vi "Write Retry on Timeout.vi"(8 "error in (no error)":errorcluster, 10 "Retry on Timeout":bool, 11 "CIFFIFO in":refnum<class "CIFfifo.lvclass">) -> (0 "error out":errorcluster, 3 "CIFFIFO out":refnum<class "CIFfifo.lvclass">)   [LabVIEW 2021, in "CIFfifo.lvclass"]
uses:
  CIFfifo.lvclass
  CIFfifo.lvclass/CIFfifo.ctl
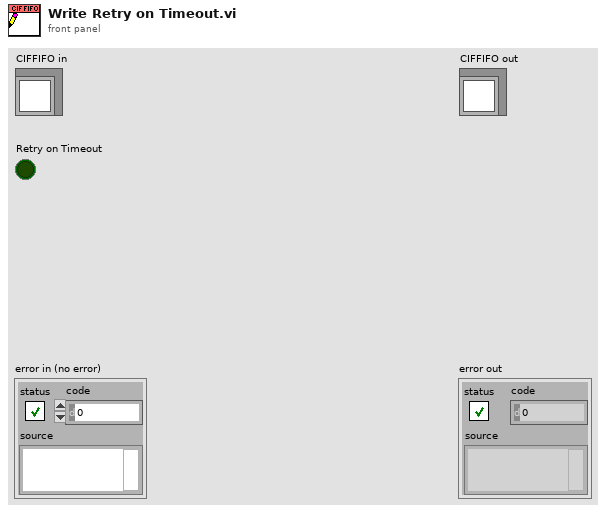
[diagram p1: front panel]
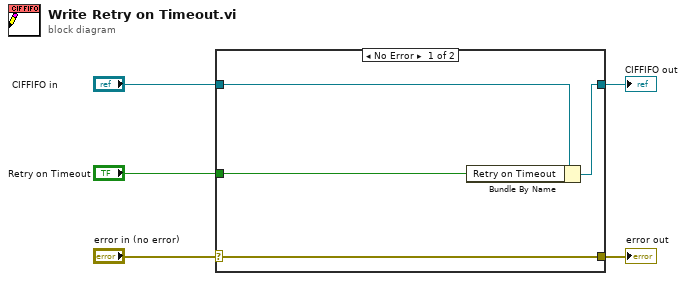
[diagram p0: block diagram]
diagram:
  n1 = case shown="No Error" "error in (no error)" {
    selector: "error in (no error)" -> [w9 w10]
    tunnel: [w9 w10] -> w4
    tunnel: [w7 w11] -> w2
    tunnel: "CIFFIFO in" -> [w8 w11]
    tunnel: "Retry on Timeout" -> [w6 _]
    frame No Error {
      n2 = Bundle By Name(cluster=w8, "Retry on Timeout"=w6) -> (w7:refnum<class "CIFfifo.lvclass">)
    }
    frame Error {
    }
  }
  "error out" <- w4
  "CIFFIFO out" <- w2
